vi "Get.vi"(7 "Pump ID (0:A)":T1, 8 "error in (no error)":errorcluster, 10 "Parameter":string, 11 "VISA resource in":refnum<visa-resource-name>) -> (0 "error out":errorcluster, 1 "Value":i32, 3 "VISA resource out":refnum<visa-resource-name>)   [LabVIEW 2020, in "Global FIA milliGAT.lvlib"]
uses:
  <instrlib>/RxnRover/Global FIA milliGAT 3.14/Global FIA milliGAT.lvlib
  <instrlib>/RxnRover/Global FIA milliGAT 3.14/Public/Utility/Pump Address.ctl
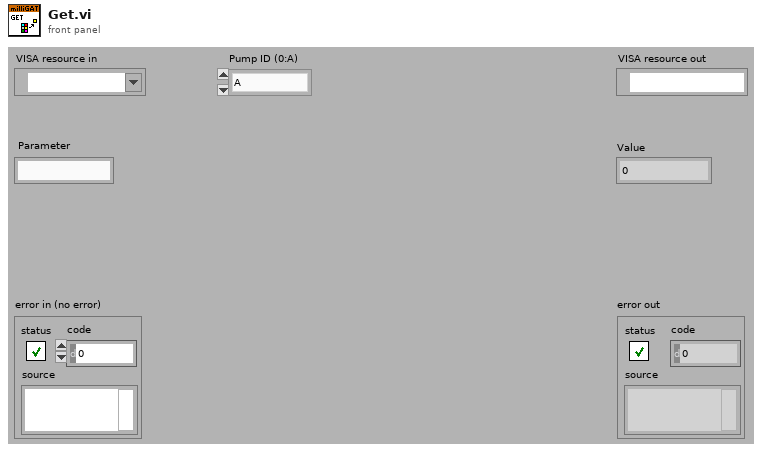
[diagram p1: front panel]
types:
  T1 = typedef "Global FIA milliGAT.lvlib/Pump Address.ctl" = enum16{"A", "B", "C", "D", "E", "F", "G", "H", "I", "J", "K", "L", "M", "N", "O", "P", "Q", "R", "S", "T", "U", "V", "W", "X", "Y", "Z", "a", "b", "c", "d", "e", "f", "g", "h", "i", "j", "k", "l", "m", "n", "o", "p", "q", "r", "s", "t", "u", "v", "w", "x", "y", "z", "0", "1", "2", "3", "4", "5", "6", "7", "8", "9"}
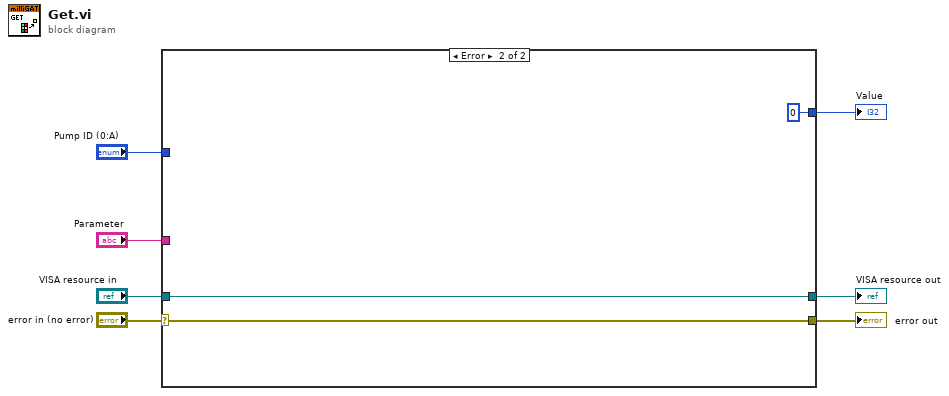
[diagram p0: block diagram]
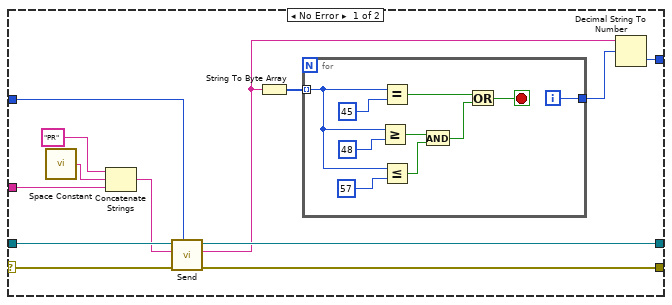
[diagram p2: hidden frame]
diagram:
  n1 = case shown="Error" "error in (no error)" {
    selector: "error in (no error)" -> [w8 w33]
    tunnel: "VISA resource in" -> [w20 w32]
    tunnel: [w19 w32] -> w6
    tunnel: "Parameter" -> [w16 _]
    tunnel: [w15 w33] -> w4
    tunnel: [w14 0] -> w3
    tunnel: "Pump ID (0:A)" -> [w13 _]
    frame No Error {
      n2 = call <vilib>:"Space Constant.vi"() -> ("String"=w17:string)
      n3 = Concatenate Strings("PR" ("string"), w17, w16) -> (w12:string)
      n4 = call <instrlib>:"Send.vi"("Pump ID (0:A)"=w13, "error in (no error)"=w8, "Command"=w12, "VISA resource in"=w20) -> ("error out"=w15:errorcluster, "Information"=w11:string, "VISA resource out"=w19:refnum<visa-resource-name>)  [unwired: 5 in]
      n5 = String To Byte Array(string=w11) -> (unsigned byte array=w10:u8[])
      n6 = for {
        tunnel: w10 -> [w27] mode=indexing
        tunnel: [w28] -> w9
        i -> [w28]
        stop <- w21 stop-if-true
        n7 = Greater Or Equal?(x=w27, y=u8 48) -> (x >= y?=w24:bool)
        n8 = Equal?(x=w27, y=u8 45) -> (x = y?=w22:bool)
        n9 = Less Or Equal?(x=w27, y=u8 57) -> (x <= y?=w25:bool)
        n10 = And(x=w24, y=w25) -> (x .and. y?=w23:bool)
        n11 = Or(x=w22, y=w23) -> (x .or. y?=w21:bool)
      }
      n12 = Decimal String To Number(string=w11, offset=w9) -> (number=w14:i32)  [unwired: 1 in, 1 out]
    }
    frame Error {
    }
  }
  "VISA resource out" <- w6
  "error out" <- w4
  "Value" <- w3
